vi "Interface Read to CRLF.vi"(8 "error in":errorcluster, 9 "timeout":i32=10000, 10 "bytes to read":i32, 11 "protocol layer in":refnum<class "Serial Interface.lvclass">) -> (0 "error out":errorcluster, 1 "timed out?":bool, 2 "data":u8[](array[numeric]), 3 "protocol layer out":refnum<class "Serial Interface.lvclass">)   [LabVIEW 2021, in "Serial Interface.lvclass"]
doc: "This provides an interface for reading from a network bus."
uses:
  Serial Interface.lvclass
  Serial Interface.lvclass/Serial Interface.ctl
  SSC/Serial Shared Components.lvlib
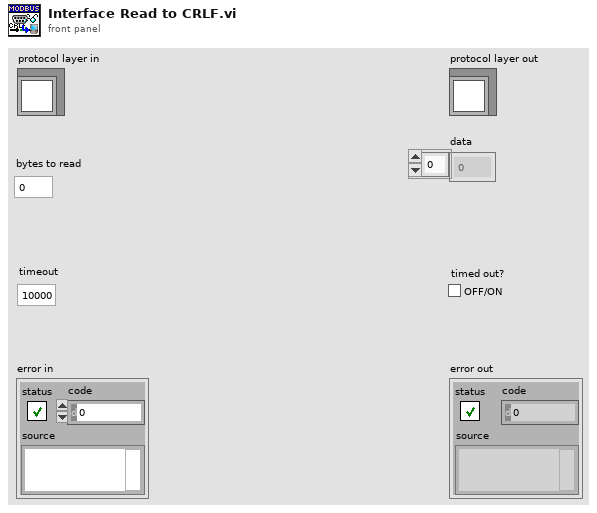
[diagram p1: front panel]
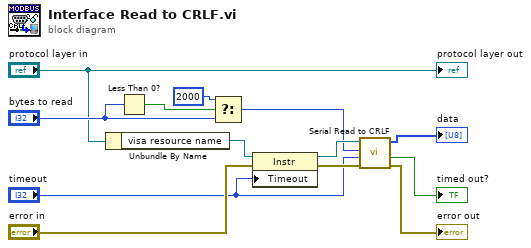
[diagram p0: block diagram]
diagram:
  n1 = Unbundle By Name("protocol layer in") -> ("visa resource name"=w10:refnum<visa-resource-name>)
  n2 = Less Than 0?(x="bytes to read") -> (x < 0?=w13:bool)
  n3 = Select(t=u32 2000, s=w13, f="bytes to read") -> (s? t:f=w1:u32)
  n4 = property class="Instr"(reference=w10, error in="error in", "Timeout"="timeout") -> (reference out=w5:refnum<visa-resource-name>, error out=w8:errorcluster)
  n5 = call "Serial Read to CRLF.vi"("error in"=w8, "timeout (ms)"="timeout", "bytes to read"=w1, "Visa Resource"=w5) -> ("error out"=→"error out":errorcluster, "timed out?"=→"timed out?":bool, "data"=→"data":u8[])  [unwired: 5 in]
  "protocol layer out" <- "protocol layer in"
